vi "HTTP_GetRequest.vi"(8 "error constant":errorcluster, 9 "output file":path=path "C:/Users/RIA/Desktop", 10 "RequestNumber":string="123456") -> (0 "error out":errorcluster, 1 "Zip path":path)   [LabVIEW 2017]
uses:
  <vilib>/httpClient/LabVIEWHTTPClient.lvlib
panel:
  out "appended path":path
  out "body":string
  out "headers":string
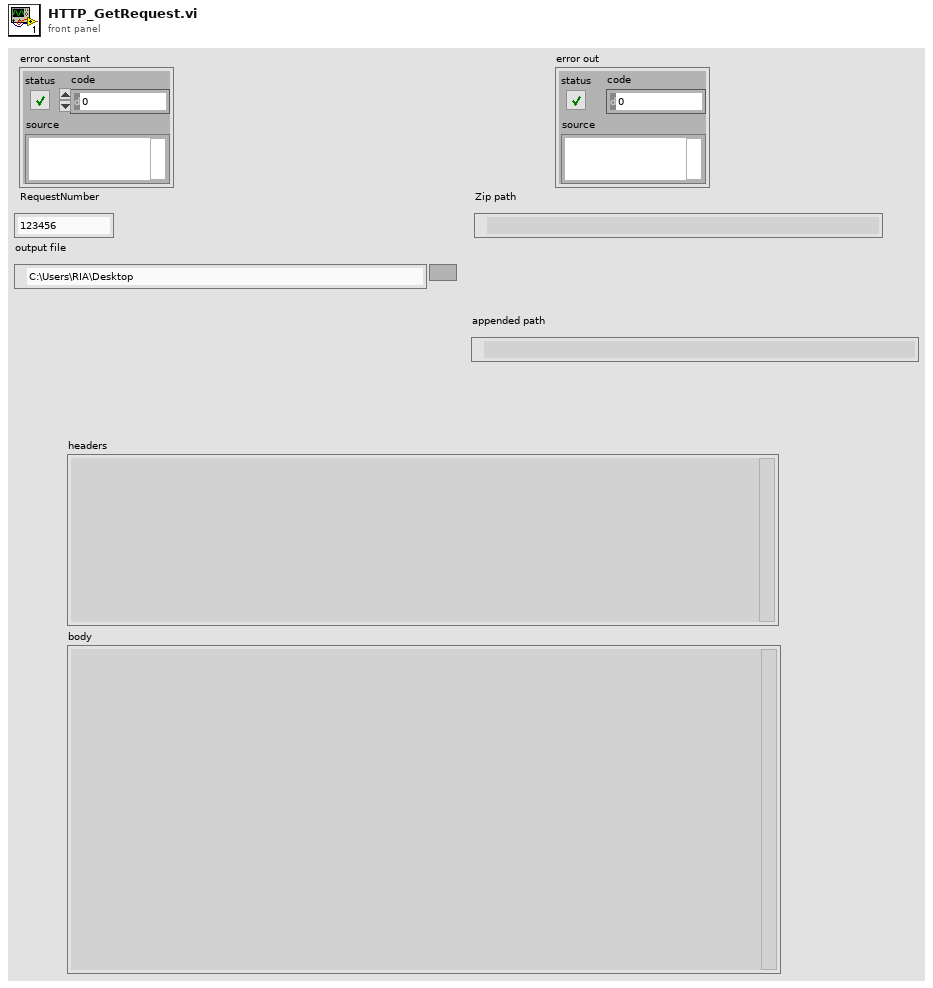
[diagram p1: front panel]
types:
  T1 = typedef "LabVIEWHTTPClient.lvlib/ClientHandle.ctl" = refnum<k1>
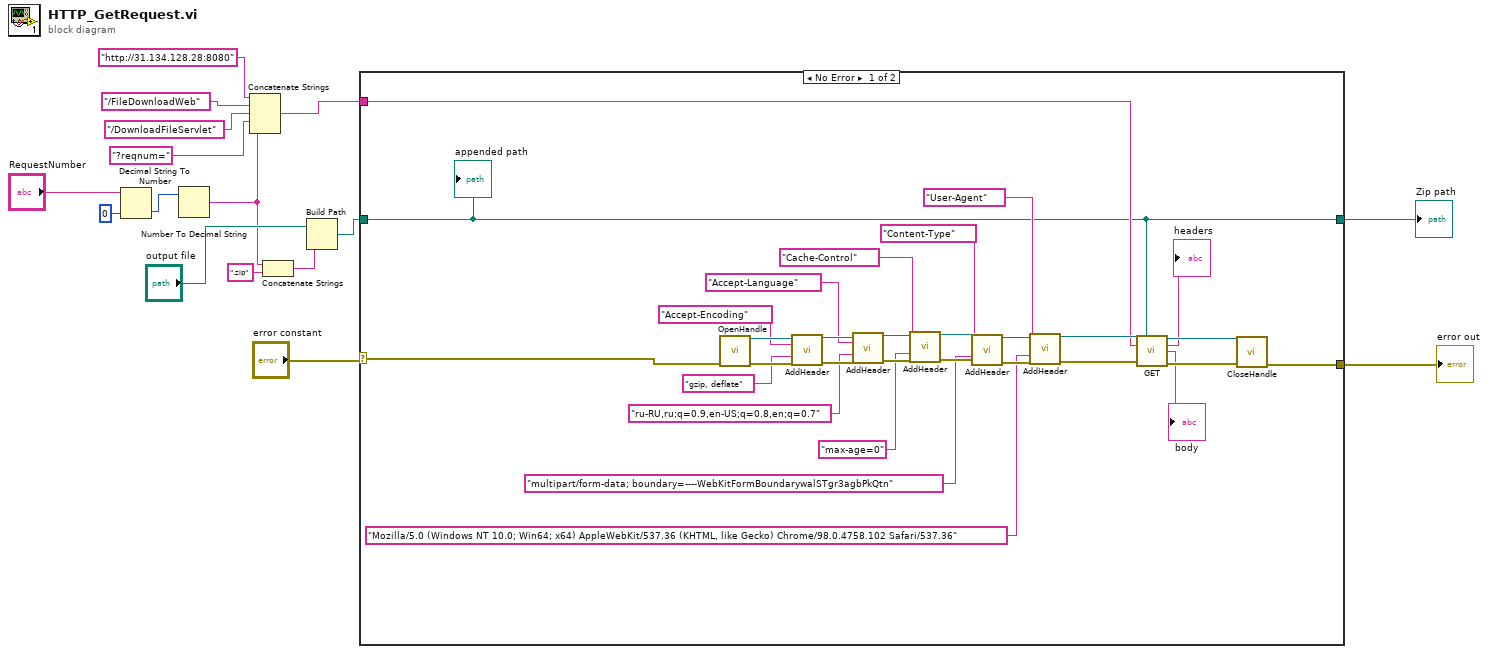
[diagram p0: block diagram]
diagram:
  n1 = Decimal String To Number(string="RequestNumber", default (0L)=i64 0 ("default (0 I32)")) -> (number=w3:i64)  [unwired: 1 in, 1 out]
  n2 = Number To Decimal String(number=w3) -> (decimal integer string=w2:string)  [unwired: 1 in]
  n3 = Concatenate Strings("http://31.134.128.28:8080" ("url"), "/FileDownloadWeb" ("url"), "/DownloadFileServlet" ("url"), "?reqnum=" ("url"), w2) -> (w13:string)
  n4 = Concatenate Strings(w2, ".zip" ("string")) -> (w6:string)
  n5 = Build Path(base path="output file", name or relative path=w6) -> (appended path=w8:path)
  n6 = case shown="No Error" "error constant" {
    selector: "error constant" -> [w29 w48]
    tunnel: [w28 w48] -> w15
    tunnel: w13 -> [w27 _]
    tunnel: w8 -> [w17 w47]
    tunnel: [w17 w47] -> w5
    frame No Error {
      n7 = call <vilib>:"OpenHandle.vi"("error in (no error)"=w29) -> ("client handle out"=w46:T1, "error out"=w41:errorcluster)  [unwired: 13 in]
      n8 = call <vilib>:"AddHeader.vi"("client handle"=w46, "header"="Accept-Encoding", "value"="gzip, deflate", "error in (no error)"=w41) -> ("client handle out"=w45:T1, "error out"=w40:errorcluster)  [unwired: 10 in]
      n9 = call <vilib>:"AddHeader.vi"("client handle"=w45, "header"="Accept-Language", "value"="ru-RU,ru;q=0.9,en-US;q=0.8,en;q=0.7", "error in (no error)"=w40) -> ("client handle out"=w44:T1, "error out"=w39:errorcluster)  [unwired: 10 in]
      n10 = call <vilib>:"AddHeader.vi"("client handle"=w44, "header"="Cache-Control", "value"="max-age=0", "error in (no error)"=w39) -> ("client handle out"=w43:T1, "error out"=w38:errorcluster)  [unwired: 10 in]
      n11 = call <vilib>:"AddHeader.vi"("client handle"=w43, "header"="Content-Type", "value"="multipart/form-data; boundary=----WebKitFormBoundarywalSTgr3agbPkQtn", "error in (no error)"=w38) -> ("client handle out"=w42:T1, "error out"=w37:errorcluster)  [unwired: 10 in]
      n12 = call <vilib>:"AddHeader.vi"("client handle"=w42, "header"="User-Agent", "value"="Mozilla/5.0 (Windows NT 10.0; Win64; x64) AppleWebKit/537.36 (KHTML, like Gecko) Chrome/98.0.4758.102 Safari/537.36", "error in (no error)"=w37) -> ("client handle out"=w36:T1, "error out"=w35:errorcluster)  [unwired: 10 in]
      n13 = call <vilib>:"GET.vi"("client handle"=w36, "output file"=w17, "url"=w27, "error in (no error)"=w35) -> ("client handle out"=w34:T1, "headers"=→"headers":string, "body"=→"body":string, "error out"=w33:errorcluster)  [unwired: 8 in]
      n14 = call <vilib>:"CloseHandle.vi"("client handle"=w34, "error in (no error)"=w33) -> ("error out"=w28:errorcluster)  [unwired: 13 in]
      "appended path" <- w17
    }
    frame Error {
    }
  }
  "error out" <- w15
  "Zip path" <- w5
